vi "Continuous Complex B-Scan Demo.vi"() -> ()   [LabVIEW 2012]
uses:
  LabVIEW/user.lib/SpectralRadar.llb/set Complex Scan Output.vi
  LabVIEW/user.lib/SpectralRadar.llb/set Apodized Spectrum Output.vi
  LabVIEW/user.lib/SpectralRadar.llb/display Data 2D.vi
  LabVIEW/user.lib/SpectralRadar.llb/OCT Device.lvclass
  LabVIEW/user.lib/SpectralRadar.llb/Probe.lvclass
  LabVIEW/user.lib/SpectralRadar.llb/Processing.lvclass
  LabVIEW/user.lib/SpectralRadar.llb/Raw Data.lvclass
  LabVIEW/user.lib/SpectralRadar.llb/Data.lvclass
  LabVIEW/user.lib/SpectralRadar.llb/Scan Pattern.lvclass
  LabVIEW/user.lib/SpectralRadar.llb/Complex Data.lvclass
panel:
  in  "stop":bool
  out "B-Scan Data":dbl[][](graph)
  out "Spectral Data":dbl[][](graph)
  in  "AScans":i32=512
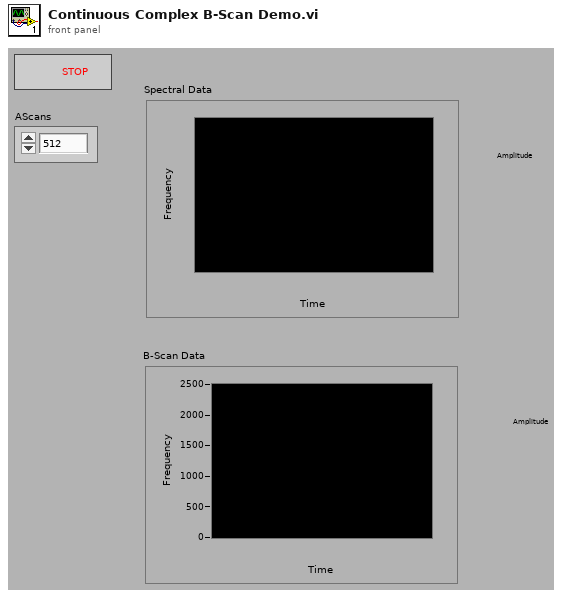
[diagram p1: front panel]
types:
  T1 = enum16{"Asynchronous Continuous", "Asynchronous Finite", "Synchronous"}
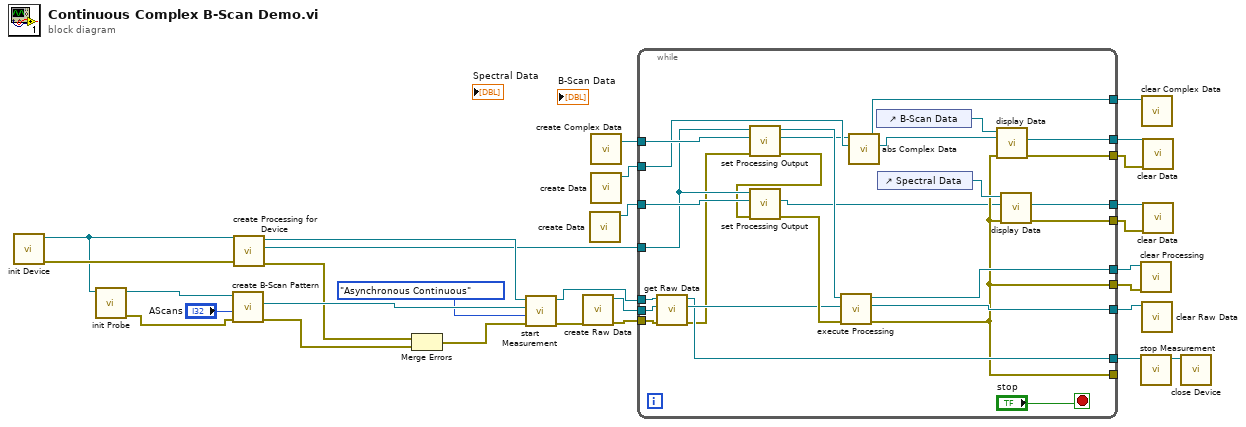
[diagram p0: block diagram]
diagram:
  n1 = call "init Device.vi"() -> ("error out"=w29:errorcluster, "OCTDevice"=w12:refnum<class "OCT Device.lvclass">)  [unwired: 6 in]
  n2 = call "init Probe.vi"("OCT Device"=w12) -> ("error out"=w11:errorcluster, "GalvoControl"=w28:refnum<class "Probe.lvclass">)  [unwired: 5 in]
  n3 = call "create B-Scan Pattern.vi"("error in (no error)"=w11, "AScans"="AScans", "Probe"=w28) -> ("error out"=w24:errorcluster, "Scan Pattern"=w26:refnum<class "Scan Pattern.lvclass">)  [unwired: 3 in, 1 out]
  n4 = call "create Processing for Device.vi"("error in (no error)"=w29, "OCTDevice"=w12) -> ("error out"=w22:errorcluster, "Processing"=w17:refnum<class "Processing.lvclass">, "OCTDevice"=w18:refnum<class "OCT Device.lvclass">)  [unwired: 3 in]
  n5 = Merge Errors(w22, w24) -> (w23:errorcluster)
  n6 = call "start Measurement.vi"("error in (no error)"=w23, "Acquisition Type"=T1."Asynchronous Continuous", "Scan Pattern"=w26, "OCTDevice"=w18) -> ("error out"=w20:errorcluster, "OCTDevice"=w8:refnum<class "OCT Device.lvclass">)  [unwired: 1 in, 1 out]
  n7 = call "create Raw Data.vi"("error in (no error)"=w20) -> ("error out"=w19:errorcluster, "Raw Data"=w21:refnum<class "Raw Data.lvclass">)  [unwired: 5 in]
  n8 = call "create Data.vi"() -> ("Data"=w2:refnum<class "Data.lvclass">)  [unwired: 6 in, 1 out]
  n9 = call "create Complex Data.vi"() -> ("Complex Data"=w16:refnum<class "Complex Data.lvclass">)  [unwired: 2 in, 1 out]
  n10 = call "create Data.vi"() -> ("Data"=w1:refnum<class "Data.lvclass">)  [unwired: 6 in, 1 out]
  n11 = while {
    tunnel: w21 -> [w55]
    tunnel: w8 -> [w56]
    tunnel: w19 -> [w54]
    tunnel: w17 -> [w51]
    tunnel: w2 -> [w53]
    tunnel: w16 -> [w52]
    tunnel: [w44] -> w15
    tunnel: [w43] -> w14
    tunnel: [w42] -> w4
    tunnel: [w41] -> w6
    tunnel: [w40] -> w3
    tunnel: [w39] -> w5
    tunnel: [w38] -> w10
    tunnel: [w36] -> w13
    tunnel: [w36] -> _
    tunnel: w1 -> [w32]
    tunnel: [w33] -> w7
    stop <- "stop" stop-if-true
    n12 = call "get Raw Data.vi"("error in (no error)"=w54, "RawData in"=w55, "OCTDevice in"=w56) -> ("error out"=w37:errorcluster, "RawData out"=w47:refnum<class "Raw Data.lvclass">, "OCTDevice out"=w38:refnum<class "OCT Device.lvclass">)  [unwired: 2 in]
    n13 = call-poly "set Processing Output.vi"("error in (no error)"=w37, "Complex Data in"=w52, "Processing"=w51) -> ("error out"=w49:errorcluster, "Complex Data out"=w31:refnum<class "Complex Data.lvclass">, "Processing"=w50:refnum<class "Processing.lvclass">)  [unwired: 2 in]
    n14 = call-poly "set Processing Output.vi"("error in (no error)"=w49, "Data"=w53, "Processing"=w51) -> ("error out"=w48:errorcluster, "Data"=w30:refnum<class "Data.lvclass">)  [unwired: 2 in, 1 out]
    n15 = call "execute Processing.vi"("error in (no error)"=w48, "Raw Data"=w47, "Processing"=w50) -> ("error out"=w36:errorcluster, "Raw Data"=w44:refnum<class "Raw Data.lvclass">, "Processing"=w43:refnum<class "Processing.lvclass">)  [unwired: 2 in]
    n16 = call "abs Complex Data.vi"("Data"=w32, "Complex Data in"=w31) -> ("Data out"=w34:refnum<class "Data.lvclass">, "Complex Data out"=w33:refnum<class "Complex Data.lvclass">)  [unwired: 3 in, 1 out]
    n17 = control-ref of="B-Scan Data"() -> (w46:refnum<vi>)
    n18 = control-ref of="Spectral Data"() -> (w45:refnum<vi>)
    n19 = call-poly "display Data.vi"("error in (no error)"=w36, "Data in"=w34, "IntGraph Refnum"=w46) -> ("error out"=w39:errorcluster, "Data out"=w41:refnum<class "Data.lvclass">)  [unwired: 2 in, 1 out]
    n20 = call-poly "display Data.vi"("error in (no error)"=w36, "Data in"=w30, "IntGraph Refnum"=w45) -> ("error out"=w40:errorcluster, "Data out"=w42:refnum<class "Data.lvclass">)  [unwired: 2 in, 1 out]
  }
  n21 = call "clear Processing.vi"("error in (no error)"=w13, "Processing"=w14) -> ()  [unwired: 5 in, 1 out]
  n22 = call "stop Measurement.vi"("OCTDevice"=w10) -> ("OCTDevice"=w9:refnum<class "OCT Device.lvclass">)  [unwired: 5 in, 1 out]
  n23 = call "clear Complex Data.vi"("Complex Data"=w7) -> ()  [unwired: 6 in, 1 out]
  n24 = call "clear Raw Data.vi"("Raw Data"=w15) -> ()  [unwired: 6 in, 1 out]
  n25 = call "clear Data.vi"("error in (no error)"=w5, "Data"=w6) -> ()  [unwired: 5 in, 1 out]
  n26 = call "clear Data.vi"("error in (no error)"=w3, "Data"=w4) -> ()  [unwired: 5 in, 1 out]
  n27 = call "close Device.vi"("OCTDevice"=w9) -> ()  [unwired: 6 in, 1 out]
